vi "Timestamp Converter.vi"() -> ()   [LabVIEW 2013]
uses:
  <vilib>/Utility/miscctls.llb/LVPointTypeDef.ctl
panel:
  in  "stop":bool
  out "Integer Time":i64
  in  "Time Stamp":timestamp
  out "time stamp":timestamp
  in  "Integer Timestamp":i64
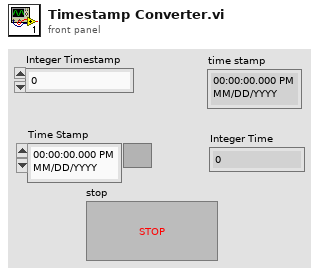
[diagram p1: front panel]
types:
  T1 = typedef "LVPointTypeDef.ctl" = cluster{"Horizontal":i16, "Vertical":i16}
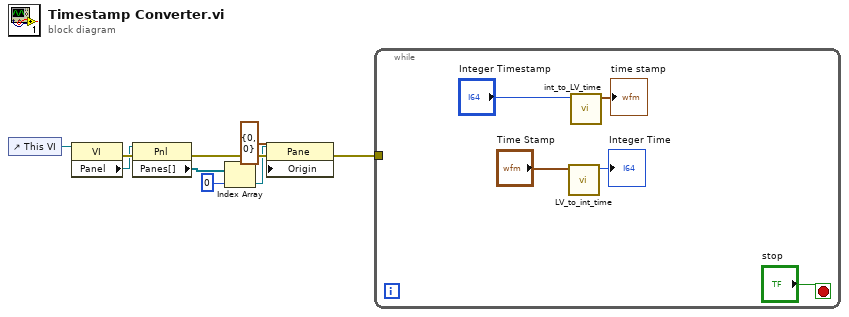
[diagram p0: block diagram]
diagram:
  n1 = control-ref of="This VI"() -> (w9:refnum<vi>)
  n2 = property class="VI"(reference=w9) -> (error out=w8:errorcluster, "Panel"=w7:refnum<vi>)  [unwired: 1 in, 1 out]
  n3 = property class="Pnl"(reference=w7, error in=w8) -> (error out=w6:errorcluster, "Panes[]"=w5:refnum<vi>[])  [unwired: 1 out]
  n4 = Index Array(array=w5, index=0) -> (element=w3:refnum<vi>)
  n5 = property class="Pane"(reference=w3, error in=w6, "Origin"=T1 {"Horizontal"=0, "Vertical"=0}) -> (error out=w1:errorcluster)  [unwired: 1 out]
  n6 = while {
    tunnel: w1 -> [_]
    stop <- "stop" stop-if-true
    n7 = call "LV_to_int_time.vi"("Time Stamp"="Time Stamp") -> ("Integer Time"=→"Integer Time":i64)  [unwired: 8 in, 1 out]
    n8 = call "int_to_LV_time.vi"("Integer Timestamp"="Integer Timestamp") -> ("time stamp"=→"time stamp":timestamp)  [unwired: 8 in, 1 out]
  }
